vi "get_Sensor_Position.vi"(8 "error in (no error)":errorcluster, 10 "Sensorkoord [P1 P2]":dbl[][](array[numeric])=[[7.0, 14.0], [0.0, 1.0]], 11 "parcour_Liste in":refnum<class "parcour_Liste.lvclass">) -> (0 "error out":errorcluster, 1 "Sensor auf Linie":bool, 2 "Schnittpunkt":dbl[](array[numeric]), 3 "parcour_Liste out":refnum<class "parcour_Liste.lvclass">)   [LabVIEW 2019, in "parcour_Liste.lvclass"]
uses:
  parcour_Liste.lvclass
  parcour_Liste.lvclass/parcour_Liste.ctl
  parcour/Parcour_element.lvclass
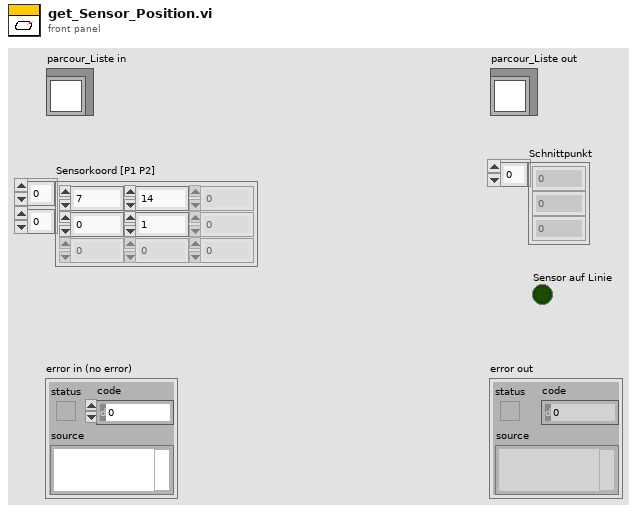
[diagram p1: front panel]
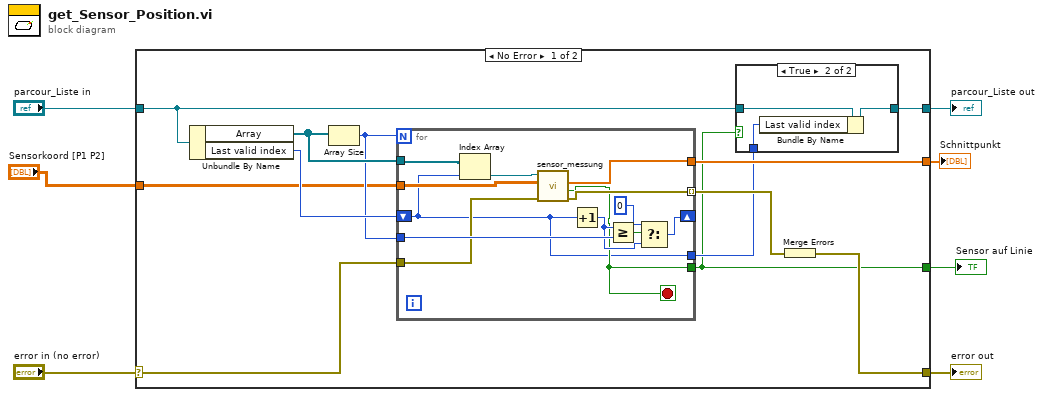
[diagram p0: block diagram]
diagram:
  n1 = case shown="No Error" "error in (no error)" {
    selector: "error in (no error)" -> [w15 w38]
    tunnel: [w13 w38] -> w6
    tunnel: [w10 w37] -> w4
    tunnel: "parcour_Liste in" -> [w19 w37]
    tunnel: "Sensorkoord [P1 P2]" -> [w12 _]
    tunnel: [w11 _] -> w2
    tunnel: [w8 _] -> w1
    frame No Error {
      n2 = Unbundle By Name(w19) -> ("Array"=w18:refnum<class "Parcour_element.lvclass">[], "Last valid index"=w17:i32)
      n3 = Array Size(array=w18) -> (size(s)=w16:i32)
      n4 = for {
        N: w16 -> [_]
        tunnel: w18 -> [w36]
        shift-right: [w31] -> _
        shift-left: w17 -> [w24]
        tunnel: w16 -> [w35]
        tunnel: w15 -> [w29]
        tunnel: [w28] -> w14 mode=indexing
        tunnel: w12 -> [w27]
        tunnel: [w26] -> w11
        tunnel: [w25] -> w8
        tunnel: [w24] -> w9
        stop <- w25 stop-if-true
        n5 = Index Array(array=w36, index=w24) -> (element=w30:refnum<class "Parcour_element.lvclass">)
        n6 = call-dynamic "sensor_messung.vi"("error in (no error)"=w29, "Sensorkoord [P1 P2]"=w27, "Parcour_element in"=w30) -> ("error out"=w28:errorcluster, "Sensor auf Linie"=w25:bool, "Schnittpunkt"=w26:dbl[])  [unwired: 5 in, 1 out]
        n7 = Increment(x=w24) -> (x+1=w33:i32)
        n8 = Greater Or Equal?(x=w33, y=w35) -> (x >= y?=w34:bool)
        n9 = Select(t=0, s=w34, f=w33) -> (s? t:f=w31:i32)
      }
      n10 = case shown="True" w8 {
        tunnel: w19 -> [w20 w23]
        tunnel: [w20 w22] -> w10
        tunnel: w9 -> [_ w21]
        frame False {
        }
        frame True {
          n11 = Bundle By Name(cluster=w23, "Last valid index"=w21) -> (w22:refnum<class "parcour_Liste.lvclass">)
        }
      }
      n12 = Merge Errors(w14) -> (w13:errorcluster)
    }
    frame Error {
    }
  }
  "error out" <- w6
  "parcour_Liste out" <- w4
  "Schnittpunkt" <- w2
  "Sensor auf Linie" <- w1
